vi "Calculate Function Query.vi"(8 "error in":errorcluster, 10 "Calculation Channel":i32(ring) items=["Calc Channel 1", "Calc Channel 2", "Calc Channel 3", "Calc Channel 4"], 11 "Instrument Handle In":i32) -> (0 "error out":errorcluster, 1 "Operation":i32, 2 "Source1":i32 caption="Source 1", 3 "Instrument Handle Out":i32, 4 "Source2":i32 caption="Source 2", 5 "Offset":dbl, 6 "Range":dbl)   [LabVIEW 8.6, in "ZTScopeM.lvlib"]
doc: "Queries the configuration of the selected calculation channel."
uses:
  ZTScopeM.lvlib
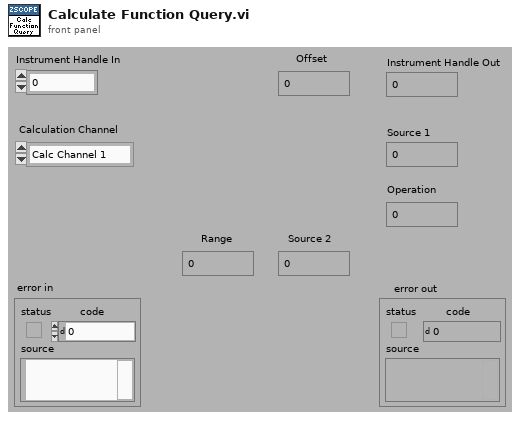
[diagram p1: front panel]
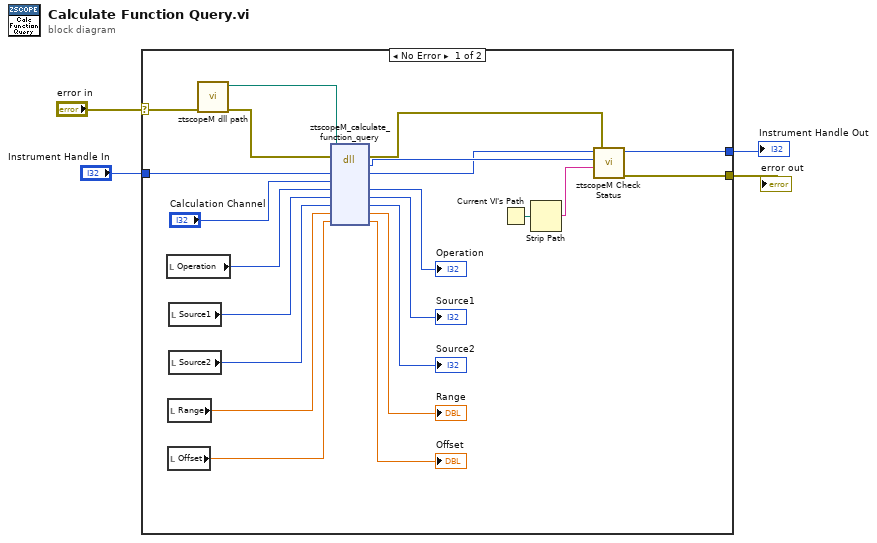
[diagram p0: block diagram]
diagram:
  n1 = case shown="No Error" "error in" {
    selector: "error in" -> [w8 w28]
    tunnel: [w10 w28] -> w2
    tunnel: "Instrument Handle In" -> [w26 w27]
    tunnel: [w9 w27] -> w3
    frame #0 {
      n2 = local read "Operation"() -> (w24:i32)
      n3 = local read "Range"() -> (w18:dbl)
      n4 = local read "Offset"() -> (w16:dbl)
      n5 = local read "Source1"() -> (w22:i32)
      n6 = local read "Source2"() -> (w20:i32)
      n7 = call "ztscopeM dll path.vi"("error in (no error)"=w8) -> ("error out"=w6:errorcluster, "<instrument>.dll path"=w7:path)  [unwired: 9 in]
      n8 = dll-call lib="C:/Program Files (x86)/National Instruments/LabVIEW 2013/instr.lib/ztscopem/ztscopeM.dll" fn="ztscopeM_calculate_function_query"(path in=w7, error in=w6, "instrumentHandle"=w26, "calculationChannel"="Calculation Channel", "operation"=w24, "source1"=w22, "source2"=w20, "range"=w18, "offset"=w16) -> (error out=w5:errorcluster, w12:i32, "instrumentHandle"=w11:i32, "operation"=→"Operation":i32, "source1"=→"Source1":i32, "source2"=→"Source2":i32, "range"=→"Range":dbl, "offset"=→"Offset":dbl)  [unwired: 2 in, 1 out]
      n9 = Current VI's Path() -> (path=w14:path)
      n10 = Strip Path(path=w14) -> (name=w13:string)  [unwired: 1 out]
      n11 = call "ztscopeM Check Status.vi"("error in"=w5, "name of VI"=w13, "status (return code)"=w12, "instrument handle in"=w11) -> ("error out"=w10:errorcluster, "instrument handle out"=w9:i32)  [unwired: 2 in]
    }
    frame #1 {
    }
  }
  "Instrument Handle Out" <- w3
  "error out" <- w2
